vi "Read bev.vi"(8 "error in (no error)":errorcluster, 11 "CondimentDecorator in":refnum<class "CondimentDecorator.lvclass">) -> (0 "error out":errorcluster, 2 "Beverage.lvclass":refnum<class "Beverage.lvclass">, 3 "CondimentDecorator out":refnum<class "CondimentDecorator.lvclass">)   [LabVIEW 2016, in "CondimentDecorator.lvclass"]
uses:
  CondimentDecorator.lvclass
  Beverage Class/Beverage.lvclass
  CondimentDecorator.lvclass/CondimentDecorator.ctl
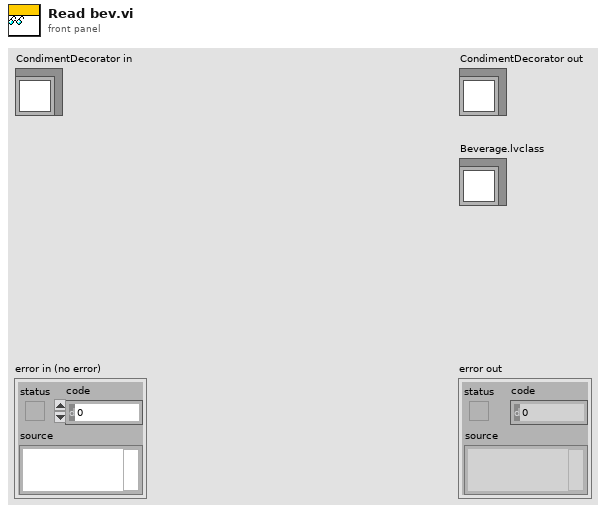
[diagram p1: front panel]
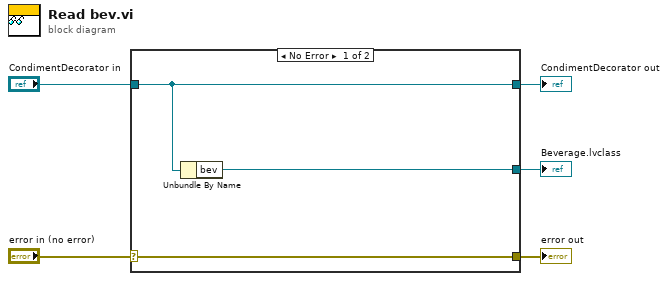
[diagram p0: block diagram]
diagram:
  n1 = case shown="No Error" "error in (no error)" {
    selector: "error in (no error)" -> [w8 w9]
    tunnel: [w8 w9] -> w4
    tunnel: [w7 w10] -> w2
    tunnel: "CondimentDecorator in" -> [w7 w10]
    tunnel: [w6 _] -> w1
    frame No Error {
      n2 = Unbundle By Name(w7) -> ("bev"=w6:refnum<class "Beverage.lvclass">)
    }
    frame Error {
    }
  }
  "error out" <- w4
  "CondimentDecorator out" <- w2
  "Beverage.lvclass" <- w1
